vi "ENPH354_A3Q1.vi"() -> ()   [LabVIEW 2020]
uses:
  <vilib>/Utility/file.llb/Read Delimited Spreadsheet (string).vi
panel:
  out "Number of Tries":u8
  in  "OK Button":bool
  in  "stop":bool
  in  "Password":string
  in  "User":string
  in  "Path":path
  # "ENPH354 Assignment 3 Q1"
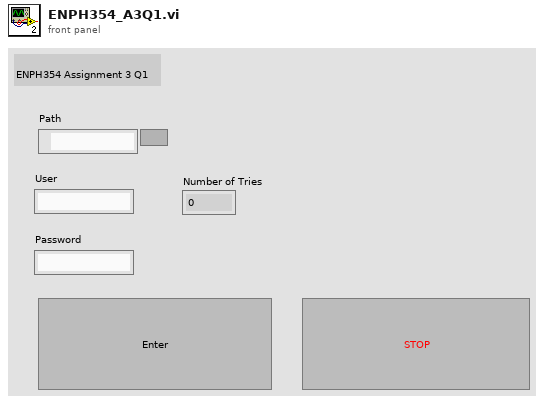
[diagram p1: front panel]
types:
  T1 = enum8{"Enabled", "Disabled", "Disabled and Grayed Out"}
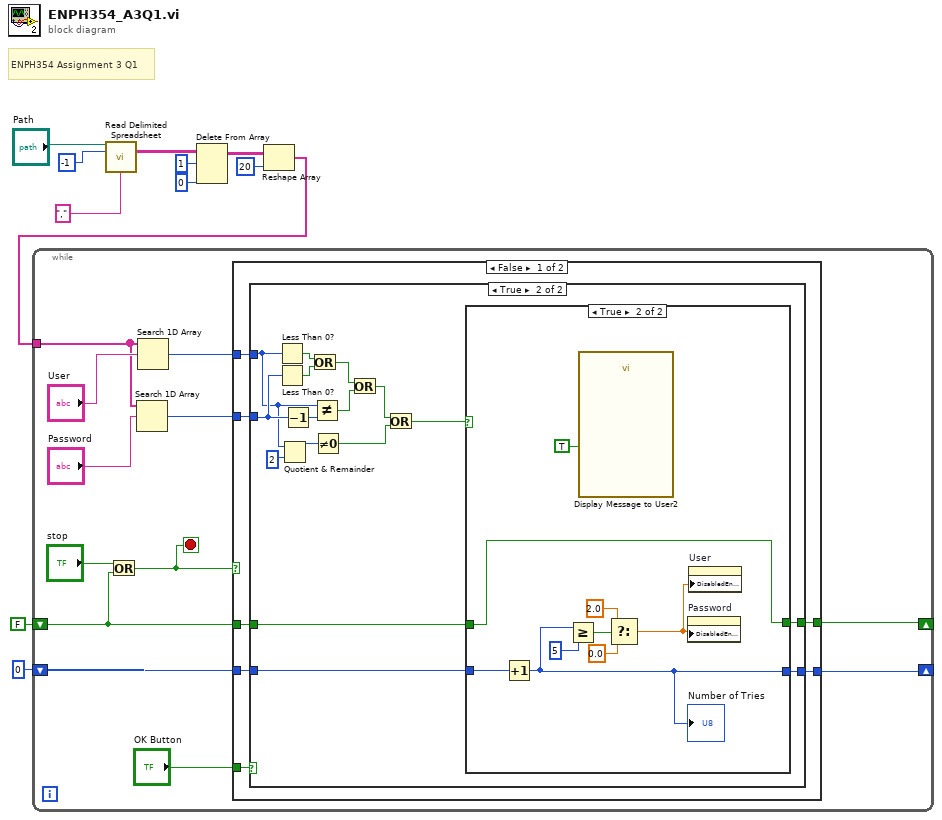
[diagram p0: block diagram]
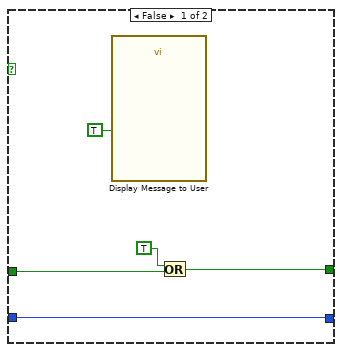
[diagram p3: hidden frame]
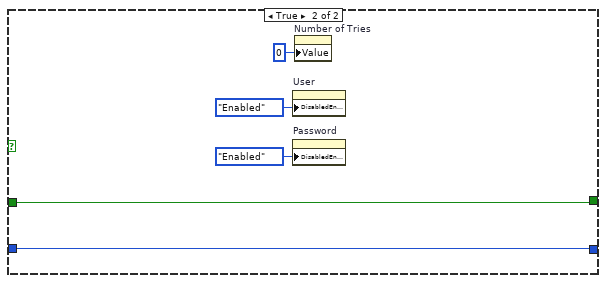
[diagram p4: hidden frame]
diagram:
  # "ENPH354 Assignment 3 Q1"
  n1 = call-poly <vilib>:"Read Delimited Spreadsheet.vi"("file path (dialog if empty)"="Path", "number of rows (all:-1)"=-1, "delimiter (\\t)"="," ("delimiter (\\t)")) -> ("all rows"=w8:string[][])  [unwired: 7 in, 5 out]
  n2 = Delete From Array(array=w8, length=1, index (row)=0) -> (array with subset deleted=w5:string[][])  [unwired: 1 in, 1 out]
  n3 = Reshape Array(w5, 20 ("dimension size")) -> (w3:string[])
  n4 = while {
    tunnel: w3 -> [w22]
    shift-right: [w13] -> _
    shift-left: 0 -> [w16]
    shift-right: [w14] -> _
    shift-left: FALSE -> [w15]
    stop <- w12 stop-if-true
    n5 = Or(x="stop", y=w15) -> (x .or. y?=w12:bool)
    n6 = Search 1D Array(1D array=w22, element="Password") -> (index of element=w18:i32)  [unwired: 1 in]
    n7 = Search 1D Array(1D array=w22, element="User") -> (index of element=w19:i32)  [unwired: 1 in]
    n8 = case shown="False" w12 {
      tunnel: w19 -> [w30 _]
      tunnel: w18 -> [w29 _]
      tunnel: "OK Button" -> [w28 _]
      tunnel: w16 -> [w27 w64]
      tunnel: w15 -> [w26 w67]
      tunnel: [w25 w67] -> w14
      tunnel: [w24 w64] -> w13
      frame False {
        n9 = case shown="True" w28 {
          tunnel: w30 -> [_ w33]
          tunnel: w29 -> [_ w39]
          tunnel: w27 -> [w31 w43]
          tunnel: [w31 w42] -> w24
          tunnel: w26 -> [w32 w41]
          tunnel: [w32 w40] -> w25
          frame False {
          }
          frame True {
            n10 = Less Than 0?(x=w33) -> (x < 0?=w47:bool)
            n11 = Less Than 0?(x=w39) -> (x < 0?=w48:bool)
            n12 = Quotient & Remainder(x=w33, y=2) -> (x-y*floor(x/y)=w37:i32)  [unwired: 1 out]
            n13 = Decrement(x=w39) -> (x-1=w46:i32)
            n14 = Or(x=w47, y=w48) -> (x .or. y?=w45:bool)
            n15 = Not Equal?(x=w33, y=w46) -> (x != y?=w44:bool)
            n16 = Not Equal To 0?(x=w37) -> (x != 0?=w35:bool)
            n17 = Or(x=w45, y=w44) -> (x .or. y?=w36:bool)
            n18 = Or(x=w36, y=w35) -> (x .or. y?=w34:bool)
            n19 = case shown="True" w34 {
              tunnel: w43 -> [w49 w56]
              tunnel: [w49 w54] -> w42
              tunnel: w41 -> [w51 w58]
              tunnel: [w50 w58] -> w40
              frame False {
                n20 = call "Display Message to User"("Enable"=TRUE) -> ()  [unwired: 9 in, 2 out]
                n21 = Or(x=TRUE, y=w51) -> (x .or. y?=w50:bool)
              }
              frame True {
                n22 = Increment(x=w56) -> (x+1=w54:i32)
                "Number of Tries" <- w54
                n23 = Greater Or Equal?(x=w54, y=5) -> (x >= y?=w61:bool)
                n24 = call "Display Message to User2"("Enable"=TRUE) -> ()  [unwired: 9 in, 2 out]
                n25 = Select(t=2.0, s=w61, f=0.0) -> (s? t:f=w57:dbl)
                n26 = property on="Password" class="Str"("DisabledEnum"=w57) -> ()  [unwired: 2 in, 2 out]
                n27 = property on="User" class="Str"("DisabledEnum"=w57) -> ()  [unwired: 2 in, 2 out]
              }
            }
          }
        }
      }
      frame True {
        n28 = property on="User" class="Str"("DisabledEnum"=T1."Enabled" ("Disabled")) -> ()  [unwired: 2 in, 2 out]
        n29 = property on="Password" class="Str"("DisabledEnum"=T1."Enabled" ("Disabled")) -> ()  [unwired: 2 in, 2 out]
        n30 = property on="Number of Tries" class="DigNum (strict)"("Value"=u8 0 ("Number of Tries")) -> ()  [unwired: 2 in, 2 out]
      }
    }
  }
